vi "Parse_Cap_Data.vi"(5 "Measure$":string, 11 "error in":errorcluster) -> (3 "CapData!":dbl format="%_6g", 4 "Capacitance Data (in pF)":dbl, 6 "Qual Data":dbl, 8 "CapFlag":dbl format="%#_13g", 10 "QualFlag":dbl format="%#_13g", 15 "error out":errorcluster)   [LabVIEW 2020]
uses:
  <vilib>/regexp/Match Regular Expression.xnode
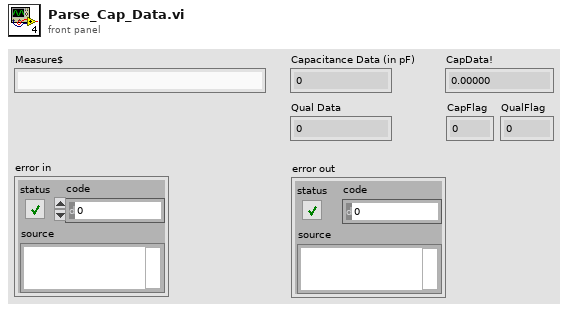
[diagram p1: front panel]
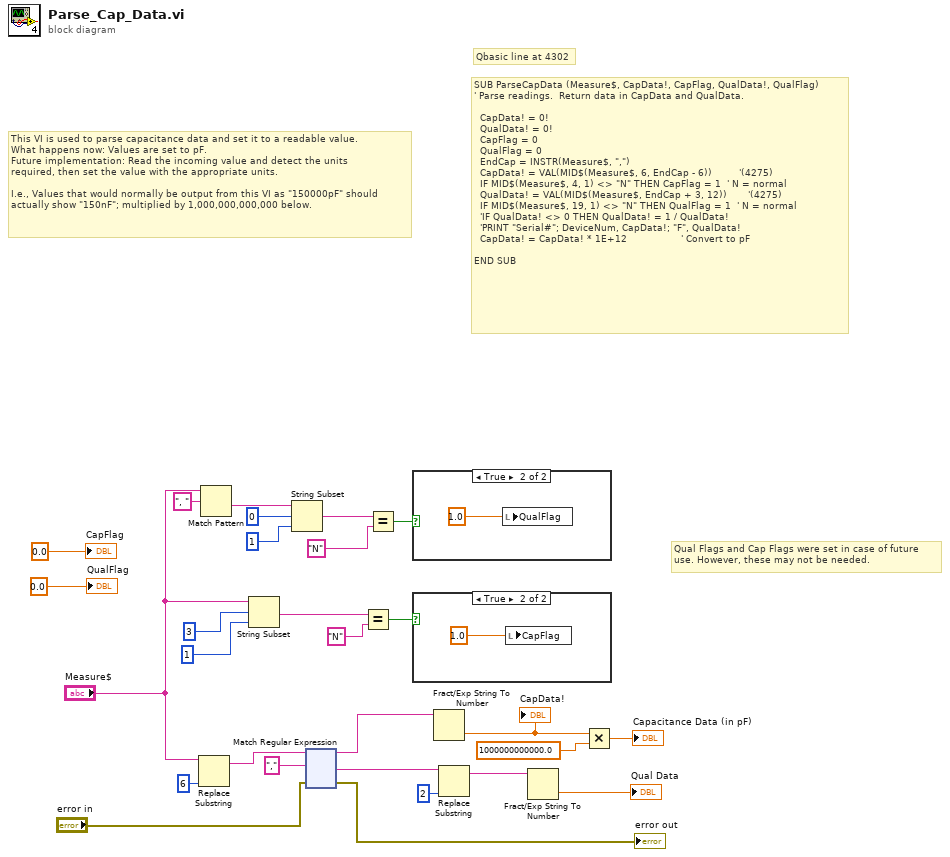
[diagram p0: block diagram]
diagram:
  # "SUB ParseCapData (Measure$, CapData!, CapFlag, QualData!, QualFlag)\n' Parse readings.  Return data in CapData and QualData.\n\n  CapData! = 0!\n  QualData! = 0!\n  CapFlag = 0\n  QualFlag = 0\n  EndCap = INSTR(Measure$, \",\")\n  CapData! = VAL(MID$(Measure$, 6, EndCap - 6))         '(4275)\n  IF MID$(Measure$, 4, 1) <> \"N\" THEN CapFlag = 1  ' N = normal\n  QualData! = VAL(MID$(Measure$, EndCap + 3, 12))       '(4275)\n  IF MID$(Measure$, 19, 1) <> \"N\" THEN QualFlag = 1  ' N = normal\n  'IF QualData! <> 0 THEN QualData! = 1 / QualData!\n  'PRINT \"Serial#\"; DeviceNum, CapData!; \"F\", QualData!\n  CapData! = CapData! * 1E+12                  ' Convert to pF\n\nEND SUB"
  # "Qbasic line at 4302"
  # "Qual Flags and Cap Flags were set in case of future\nuse. However, these may not be needed."
  # "This VI is used to parse capacitance data and set it to a readable value.\nWhat happens now: Values are set to pF.\nFuture implementation: Read the incoming value and detect the units\nrequired, then set the value with the appropriate units.\n\nI.e., Values that would normally be output from this VI as \"150000pF\" should\nactually show \"150nF\"; multiplied by 1,000,000,000,000 below."
  n1 = Replace Substring(2:6 ("length (len. of substring)"), 5:"Measure$") -> (1:w4:string)  [unwired: 2 in, 1 out]
  n2 = Match Pattern(string="Measure$", regular expression=", ") -> (after substring=w11:string)  [unwired: 1 in, 3 out]
  n3 = String Subset(string="Measure$", offset (0)=3, length (rest)=1 ("length (rest)")) -> (substring=w15:string)
  n4 = String Subset(string=w11, offset (0)=0, length (rest)=1 ("length (rest)")) -> (substring=w8:string)
  n5 = xnode "Match Regular Expression"("input string"=w4, "regular expression"=",", "error in"="error in") -> ("before match"=w22:string, "after match"=w3:string, "error out"=→"error out":errorcluster)  [unwired: 3 in, 2 out]
  n6 = Equal?(x=w15, y="N") -> (x = y?=w20:bool)
  n7 = Equal?(x=w8, y="N") -> (x = y?=w13:bool)
  n8 = case shown="True" w13 {
    frame False {
    }
    frame True {
      n9 = local write "QualFlag"(1.0) -> ()
    }
  }
  n10 = case shown="True" w20 {
    frame False {
    }
    frame True {
      n11 = local write "CapFlag"(1.0) -> ()
    }
  }
  n12 = Fract/Exp String To Number(string=w22) -> (number=w24:dbl)  [unwired: 3 in, 1 out]
  "CapData!" <- w24
  n13 = Replace Substring(2:2 ("length (len. of substring)"), 5:w3) -> (1:w2:string)  [unwired: 2 in, 1 out]
  n14 = Fract/Exp String To Number(string=w2) -> (number=→"Qual Data":dbl)  [unwired: 3 in, 1 out]
  n15 = Multiply(x=w24, y=1000000000000.0) -> (x*y=→"Capacitance Data (in pF)":dbl)
  "CapFlag" <- 0.0
  "QualFlag" <- 0.0
